vi "Init Msg.vi"(6 "Teller":refnum<class "Teller.lvclass">, 9 "Error":errorcluster, 10 "Actor":refnum<class "Actor.lvclass">) -> (3 "Stopped Msg out":refnum<class "--Stopped Msg.lvclass">)   [LabVIEW 2025, in "jettl.lvlib" / "Stopped jettl Msg.lvlib" / "--Stopped Msg.lvclass"]
uses:
  --Stopped Msg.lvclass
  Actor/Actor.lvclass
  Teller/Teller.lvclass
  --Stopped Msg.lvclass/--Stopped Msg.ctl
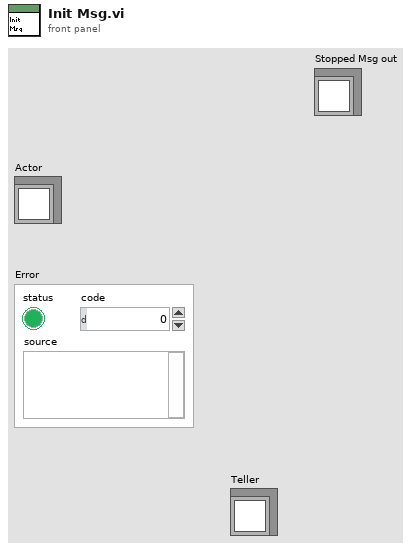
[diagram p1: front panel]
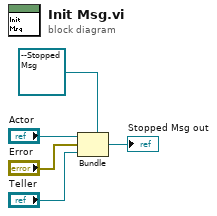
[diagram p0: block diagram]
diagram:
  n1 = Bundle "Bundle"(cluster=refnum<class "--Stopped Msg.lvclass"> refnum ("Last Ack Creator Queue Msg Strategy out"), "Actor", "Error", "Teller") -> (→"Stopped Msg out":refnum<class "--Stopped Msg.lvclass">)
